vi "ReadBomb.vi"(8 "error in (no error)":errorcluster, 11 "BombedWall":refnum<class "BombedWall.lvclass">) -> (0 "error out":errorcluster, 2 "bomb":bool, 3 "BombedWall":refnum<class "BombedWall.lvclass">)   [LabVIEW 2020, in "BombedWall.lvclass"]
uses:
  BombedWall.lvclass
  BombedWall.lvclass/BombedWall.ctl
  TypeDef/privateDataDVR.ctl
  TypeDef/privateData.ctl
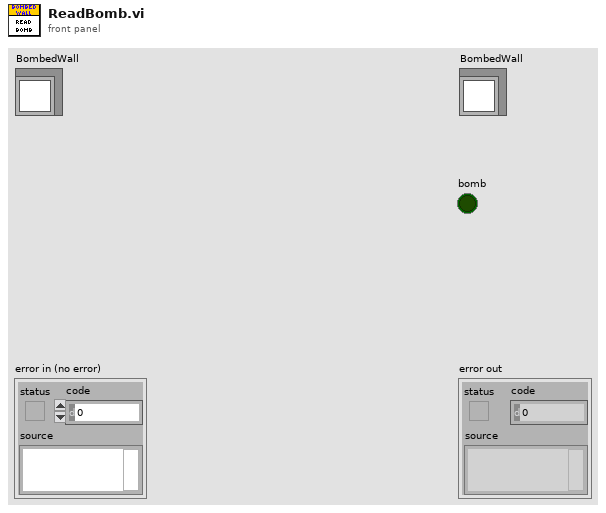
[diagram p1: front panel]
types:
  T1 = typedef "BombedWall.lvclass/privateDataDVR.ctl" = refnum<data-value>
  T2 = typedef "BombedWall.lvclass/privateData.ctl" = cluster{"bomb":bool}
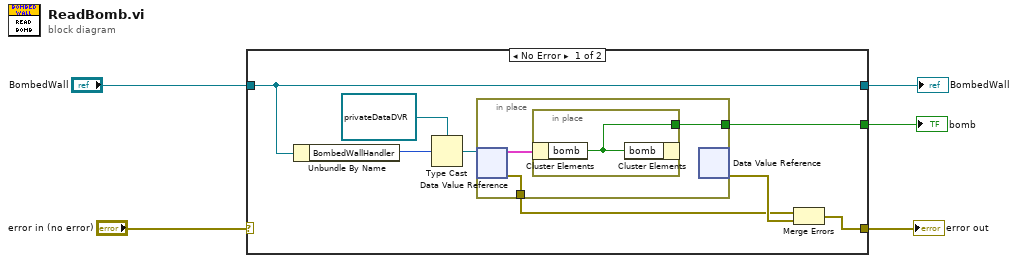
[diagram p0: block diagram]
diagram:
  n1 = case shown="No Error" "error in (no error)" {
    selector: "error in (no error)" -> [_ w18]
    tunnel: "BombedWall" -> [w13 w19]
    tunnel: [w13 w19] -> w4
    tunnel: [w12 w18] -> w1
    tunnel: [w7 _] -> w3
    frame No Error {
      n2 = Unbundle By Name(w13) -> ("BombedWallHandler"=w8:u32)
      n3 = Type Cast(type=T1 refnum ("privateDataDVR"), x=w8) -> (*(type *) &x=w10:T1)
      n4 = in-place {
        in-place-border: [w15] -> w7
        in-place-border: [w14] -> w6
        n5 = in-place-dvr #1(w10) -> (w16:T2, w14:errorcluster)
        n6 = in-place {
          in-place-border: [w17] -> w15
          n7 = in-place-cluster #2(w16) -> ("bomb"=w17:bool)
          n8 = in-place-cluster #2("bomb"=w17) -> ()  [unwired: 1 out]
        }
        n9 = in-place-dvr #1() -> (w9:errorcluster)  [unwired: 1 in, 1 out]
      }
      n10 = Merge Errors(w6, w9) -> (w12:errorcluster)
    }
    frame Error {
    }
  }
  "error out" <- w1
  "BombedWall" <- w4
  "bomb" <- w3
